vi "Downhill Simplex nD Inner Part.vi"(6 "Parsed Formula":cluster{"Table":i32[][], "Y Values":dbl[]}, 7 "Variables":i32[](array[numeric]), 9 "accuracy":dbl format="%.2f", 10 "f(Minimum) before":dbl[](array[numeric]) format="%.2f", 11 "Minimum before":dbl[][](array[numeric]) format="%.2f") -> (2 "f(Minimum) after":dbl[](array[numeric]) format="%.2f", 3 "Minimum after":dbl[][](array[numeric]) format="%.2f", 4 "convergence":bool)   [LabVIEW 2018, in "NI_Gmath.lvlib"]
uses:
  NI_Gmath.lvlib
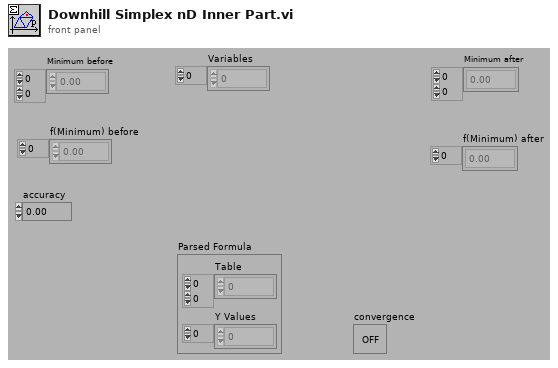
[diagram p1: front panel]
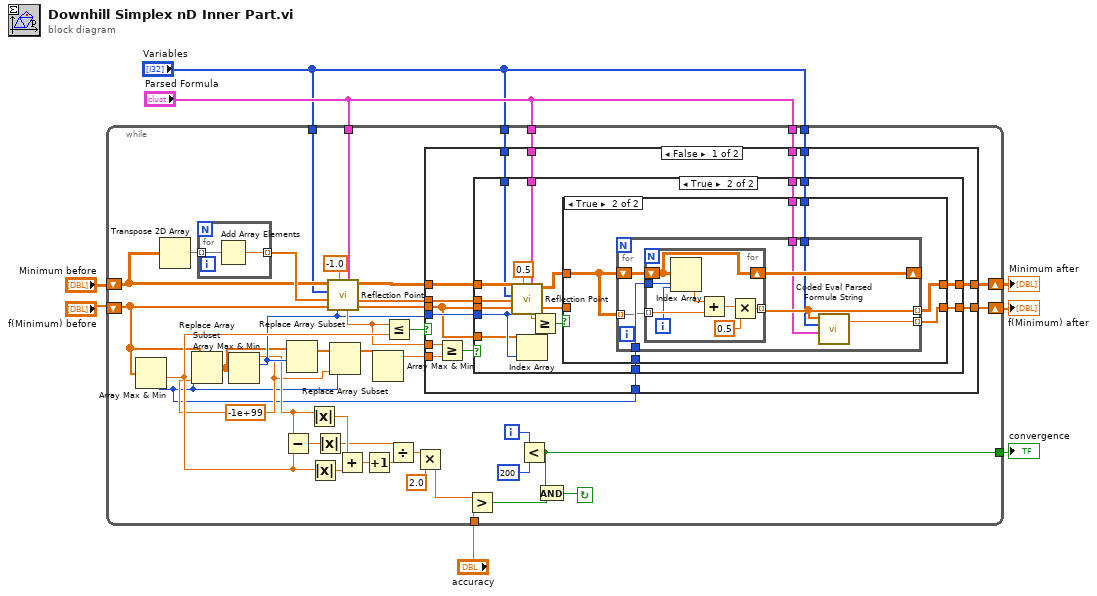
[diagram p0: block diagram]
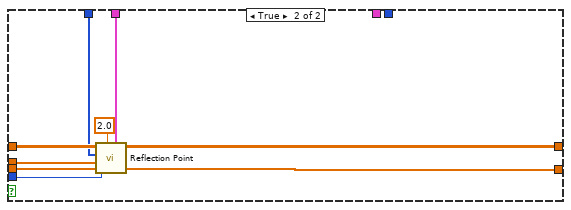
[diagram p4: hidden frame]
diagram:
  n1 = while {
    tunnel: [w17] -> w7
    tunnel: "accuracy" -> [w42]
    shift-left: "f(Minimum) before" -> [w28]
    shift-right: [w21] -> w6
    shift-left: "Minimum before" -> [w15]
    shift-right: [w22] -> w4
    tunnel: "Parsed Formula" -> [w12]
    tunnel: "Variables" -> [w11]
    tunnel: "Parsed Formula" -> [w13]
    tunnel: "Variables" -> [w14]
    tunnel: "Parsed Formula" -> [w10]
    tunnel: "Variables" -> [w9]
    i -> [w20]
    stop <- w16 continue-if-true
    w26 = -1e+99
    n2 = Array Max & Min(array=w28) -> (min value=w41:dbl, min index (indices)=w25:i32)  [unwired: 2 out]
    n3 = Transpose 2D Array(2D array=w15) -> (transposed array=w50:dbl[][])
    n4 = Replace Array Subset(array=w28, new element=w26, index=w25) -> (w27:dbl[])
    n5 = for {
      tunnel: w50 -> [w119] mode=indexing
      tunnel: [w118] -> w38 mode=indexing
      n6 = Add Array Elements(numeric array=w119) -> (sum=w118:dbl)
    }
    n7 = Array Max & Min(array=w27) -> (max value=w29:dbl, max index (indices)=w30:i32)  [unwired: 2 out]
    n8 = Subtract(x=w29, y=w41) -> (x-y=w49:dbl)
    n9 = Replace Array Subset(array=w27, new element=w26, index=w30) -> (w32:dbl[])
    n10 = Absolute Value(x=w29) -> (abs(x)=w48:dbl)
    n11 = Absolute Value(x=w41) -> (abs(x)=w47:dbl)
    n12 = Absolute Value(x=w49) -> (abs(x)=w46:dbl)
    n13 = call "Reflection Point.vi"("Parsed Formula"=w12, "high index"=w30, "factor"=-1.0, "f values before"=w28, "psum before"=w38, "Variables"=w11, "points before"=w15) -> ("f values after"=w35:dbl[], "psum after"=w36:dbl[], "points after"=w37:dbl[][], "new f value"=w34:dbl)  [unwired: 1 in]
    n14 = Replace Array Subset(array=w32, new element=w26, index=w25) -> (w31:dbl[])
    n15 = Add(x=w48, y=w47) -> (x+y=w45:dbl)
    n16 = Increment(x=w45) -> (x+1=w23:dbl)
    n17 = Array Max & Min(array=w31) -> (max value=w33:dbl)  [unwired: 3 out]
    n18 = Less Or Equal?(x=w34, y=w41) -> (x <= y?=w40:bool)
    n19 = Divide(x=w46, y=w23) -> (x/y=w44:dbl)
    n20 = Multiply(x=w44, y=2.0) -> (x*y=w24:dbl)
    n21 = case shown="False" w40 {
      tunnel: w37 -> [w61 w116]
      tunnel: w36 -> [w60 w115]
      tunnel: w35 -> [w55 w114]
      tunnel: w30 -> [w59 w113]
      tunnel: [w57 w112] -> w22
      tunnel: [w56 w111] -> w21
      tunnel: w34 -> [w64 _]
      tunnel: w33 -> [w63 _]
      tunnel: w25 -> [w58 _]
      tunnel: w14 -> [w54 _]
      tunnel: w13 -> [w53 _]
      tunnel: w10 -> [w52 w110]
      tunnel: w9 -> [w51 w109]
      frame False {
        n22 = Greater Or Equal?(x=w64, y=w63) -> (x >= y?=w62:bool)
        n23 = case shown="True" w62 {
          tunnel: w61 -> [w66 w83]
          tunnel: w60 -> [_ w82]
          tunnel: w55 -> [w65 w81]
          tunnel: w59 -> [_ w73]
          tunnel: w58 -> [_ w78]
          tunnel: [w66 w76] -> w57
          tunnel: [w65 w75] -> w56
          tunnel: w55 -> [_ w72]
          tunnel: w54 -> [_ w70]
          tunnel: w53 -> [_ w69]
          tunnel: w52 -> [_ w68]
          tunnel: w51 -> [_ w67]
          frame False {
          }
          frame True {
            n24 = call "Reflection Point.vi"("Parsed Formula"=w68, "high index"=w73, "factor"=0.5, "f values before"=w81, "psum before"=w82, "Variables"=w67, "points before"=w83) -> ("f values after"=w74:dbl[], "points after"=w77:dbl[][], "new f value"=w80:dbl)  [unwired: 1 in, 1 out]
            n25 = Index Array(array=w72, index=w73) -> (element=w71:dbl)
            n26 = Greater Or Equal?(x=w80, y=w71) -> (x >= y?=w79:bool)
            n27 = case shown="True" w79 {
              tunnel: w78 -> [_ w92]
              tunnel: w77 -> [w86 w89]
              tunnel: [w86 w91] -> w76
              tunnel: [w85 w90] -> w75
              tunnel: w74 -> [w85 _]
              tunnel: w70 -> [_ w88]
              tunnel: w69 -> [_ w87]
              frame False {
              }
              frame True {
                n28 = for {
                  tunnel: w92 -> [w98]
                  shift-right: [w99] -> _
                  shift-left: w89 -> [w100]
                  tunnel: w89 -> [w97] mode=indexing
                  tunnel: [w95] -> w91 mode=indexing
                  tunnel: [w96] -> w90 mode=indexing
                  tunnel: w88 -> [w94]
                  tunnel: w87 -> [w93]
                  n29 = for {
                    shift-right: [w103] -> w99
                    shift-left: w100 -> [w103]
                    tunnel: w98 -> [w101]
                    tunnel: w97 -> [w108] mode=indexing
                    tunnel: [w104] -> w95 mode=indexing
                    i -> [w102]
                    n30 = Index Array(array=w103, index (row)=w101, index (col)=w102) -> (element=w107:dbl)
                    n31 = Add(x=w107, y=w108) -> (x+y=w106:dbl)
                    n32 = Multiply(x=w106, y=0.5) -> (x*y=w104:dbl)
                  }
                  n33 = call "Coded Eval Parsed Formula String.vi"("Parsed Formula"=w93, "Variables"=w94, "X Values"=w95) -> ("y value"=w96:dbl)  [unwired: 1 in, 1 out]
                }
              }
            }
          }
        }
      }
      frame True {
        n34 = call "Reflection Point.vi"("Parsed Formula"=w110, "high index"=w113, "factor"=2.0, "f values before"=w114, "psum before"=w115, "Variables"=w109, "points before"=w116) -> ("f values after"=w111:dbl[], "points after"=w112:dbl[][])  [unwired: 1 in, 2 out]
      }
    }
    n35 = Greater?(x=w24, y=w42) -> (0:w18:bool)
    n36 = Less?(x=w20, y=200) -> (x < y?=w17:bool)
    n37 = And(x=w17, y=w18) -> (x .and. y?=w16:bool)
  }
  "convergence" <- w7
  "f(Minimum) after" <- w6
  "Minimum after" <- w4
